vi "Convert Annulus to ROI for Overlay.vi"(8 "error in (no error)":errorcluster, 11 "Mask ROI In":T1={"left annulus"={"Center X"=929, "Center Y"=663, "Inner Radius"=200, "Outer Radius"=405, "Start Angle"=90.0, "End Angle"=180.0}, "right annulus"={"Center X"=929, "Center Y"=663, "Inner Radius"=200, "Outer Radius"=405, "Start Angle"=90.0, "End Angle"=180.0}, "Threshold Range"={"Lower value"=106.82432432432432, "Upper value"=255.0}, "[Avg BG]"=[], "Number of Sectors"=0, "Left ROI"={"Global Rectangle"=[], "Contours"=[]}, "Right ROI"={"Global Rectangle"=[], "Contours"=[]}, "Left Start Angle Duty Cycle"=0.0, "Left End Angle Duty Cycle"=0.0, "Right End Angle Duty Cycle"=0.0, "Right Start Angle Duty Cycle"=0.0, "[Sector ROIs]"=[], "Consecutive Sector Threshold"=0} {"[Sector ROIs]"."Contours"."Type" items=["No Selection", "Point", "Line", "Rectangle", "Oval", "Polygon", "Freehand Region", "Annulus", "Unused2", "Unused3", "Broken Line", "Freehand Line", "Rotated Rectangle"]; "Right ROI"."Contours"."Type" items=["No Selection", "Point", "Line", "Rectangle", "Oval", "Polygon", "Freehand Region", "Annulus", "Unused2", "Unused3", "Broken Line", "Freehand Line", "Rotated Rectangle"]; "Left ROI"."Contours"."Type" items=["No Selection", "Point", "Line", "Rectangle", "Oval", "Polygon", "Freehand Region", "Annulus", "Unused2", "Unused3", "Broken Line", "Freehand Line", "Rotated Rectangle"]; "Threshold Range"."Upper value" min=0.0 max=255.0 scale=0.0..255.0; "Threshold Range"."Lower value" min=0.0 max=255.0 scale=0.0..255.0; "right annulus"."End Angle" format="%.2f"; "right annulus"."Start Angle" format="%.2f"; "right annulus"."Center X" scale=0.0..1024.0; "left annulus"."End Angle" format="%.2f"; "left annulus"."Start Angle" format="%.2f"; "left annulus"."Center X" scale=0.0..1024.0}) -> (0 "error out":errorcluster, 3 "Mask ROI Out":T1={"left annulus"={"Center X"=929, "Center Y"=663, "Inner Radius"=200, "Outer Radius"=405, "Start Angle"=90.0, "End Angle"=180.0}, "right annulus"={"Center X"=929, "Center Y"=663, "Inner Radius"=200, "Outer Radius"=405, "Start Angle"=90.0, "End Angle"=180.0}, "Threshold Range"={"Lower value"=106.82432432432432, "Upper value"=255.0}, "[Avg BG]"=[0, 0, 0, 0, 0, 0, 0, 0, 0, 0, 0, 0, 0, 0, 0, 0, 0, 0, 0, 0, 0, 0, 0, 0, 0, 0, 0, 0, 0, 0, 0, 0], "Number of Sectors"=0, "Left ROI"={"Global Rectangle"=[], "Contours"=[]}, "Right ROI"={"Global Rectangle"=[], "Contours"=[]}, "Left Start Angle Duty Cycle"=0.0, "Left End Angle Duty Cycle"=0.0, "Right End Angle Duty Cycle"=0.0, "Right Start Angle Duty Cycle"=0.0, "[Sector ROIs]"=[], "Consecutive Sector Threshold"=0} {"[Sector ROIs]"."Contours"."Type" items=["No Selection", "Point", "Line", "Rectangle", "Oval", "Polygon", "Freehand Region", "Annulus", "Unused2", "Unused3", "Broken Line", "Freehand Line", "Rotated Rectangle"]; "Right ROI"."Contours"."Type" items=["No Selection", "Point", "Line", "Rectangle", "Oval", "Polygon", "Freehand Region", "Annulus", "Unused2", "Unused3", "Broken Line", "Freehand Line", "Rotated Rectangle"]; "Left ROI"."Contours"."Type" items=["No Selection", "Point", "Line", "Rectangle", "Oval", "Polygon", "Freehand Region", "Annulus", "Unused2", "Unused3", "Broken Line", "Freehand Line", "Rotated Rectangle"]; "Threshold Range"."Upper value" min=0.0 max=255.0 scale=0.0..255.0; "Threshold Range"."Lower value" min=0.0 max=255.0 scale=0.0..255.0; "right annulus"."End Angle" format="%.2f"; "right annulus"."Start Angle" format="%.2f"; "right annulus"."Center X" scale=0.0..1024.0; "left annulus"."End Angle" format="%.2f"; "left annulus"."Start Angle" format="%.2f"; "left annulus"."Center X" scale=0.0..1024.0})   [LabVIEW 2013]
uses:
  Image Processing/Mask ROI Cluster.ctl
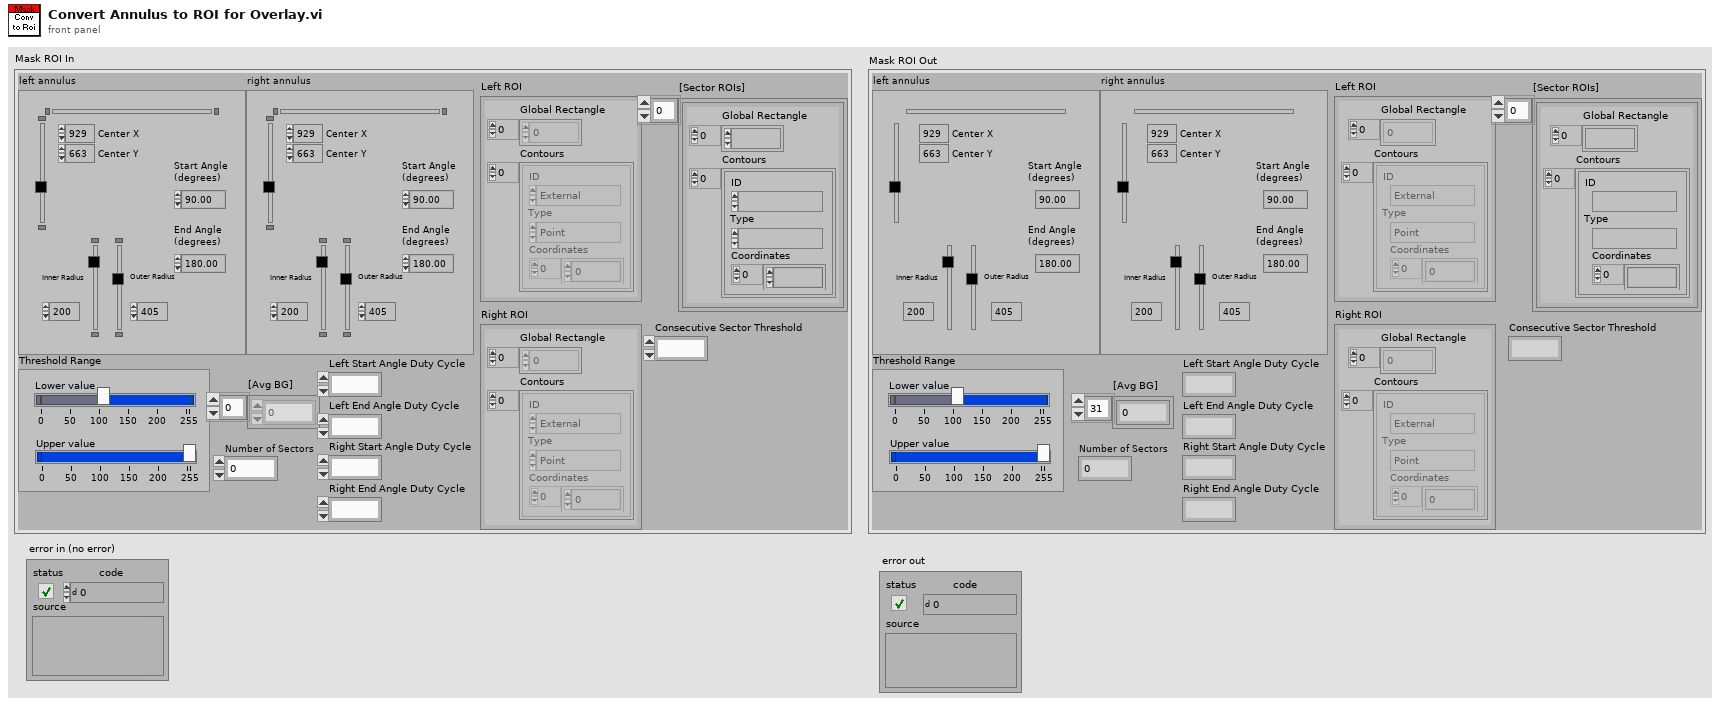
[diagram p1: front panel]
types:
  T1 = typedef "Mask ROI Cluster.ctl" = cluster{"left annulus":T2, "right annulus":T2, "Threshold Range":cluster{"Lower value":dbl, "Upper value":dbl}, "[Avg BG]":u8[], "Number of Sectors":u8, "Left ROI":T3, "Right ROI":T3, "Left Start Angle Duty Cycle":fxp<+,8,0>, "Left End Angle Duty Cycle":fxp<+,8,0>, "Right End Angle Duty Cycle":fxp<+,8,0>, "Right Start Angle Duty Cycle":fxp<+,8,0>, "[Sector ROIs]":T3[], "Consecutive Sector Threshold":u8}
  T2 = typedef "IMAQ Circle" = cluster{"Center X":i32, "Center Y":i32, "Inner Radius":i32, "Outer Radius":i32, "Start Angle":dbl, "End Angle":dbl}
  T3 = typedef "ROI Descriptor" = cluster{"Global Rectangle":i32[], "Contours":cluster{"ID":enum32{"External", "Internal"}, "Type":u32, "Coordinates":i32[]}[]}
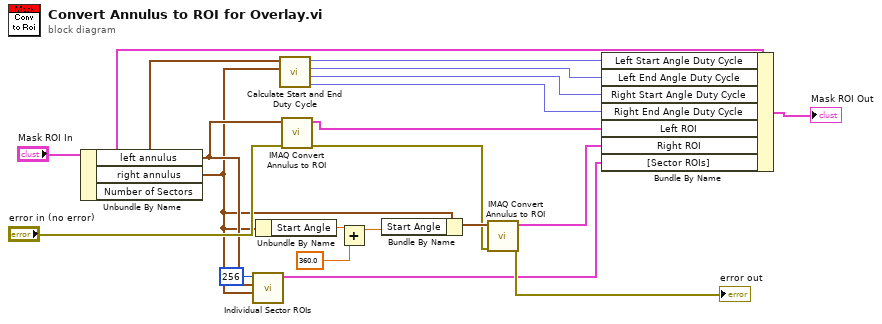
[diagram p0: block diagram]
diagram:
  n1 = Unbundle By Name("Mask ROI In") -> ("left annulus"=w3:T2, "right annulus"=w2:T2)  [unwired: 1 out]
  n2 = call "Individual Sector ROIs.vi"("right annulus"=w2, "left annulus"=w3, "Number of Sectors"=u16 256) -> ("Sector ROIs"=w4:T3[])  [unwired: 8 in]
  n3 = Unbundle By Name(w2) -> ("Start Angle"=w19:dbl)
  n4 = call "Calculate Start and End Duty Cycle.vi"("right annulus"=w2, "left annulus"=w3) -> ("Right End Angle Duty Cycle"=w5:fxp<+,8,0>, "Right Start Angle Duty Cycle"=w6:fxp<+,8,0>, "Left End Angle Duty Cycle"=w7:fxp<+,8,0>, "Left Start Angle Duty Cycle"=w8:fxp<+,8,0>)  [unwired: 6 in]
  n5 = call "IMAQ Convert Annulus to ROI"("error in (no error)"="error in (no error)", "Annulus"=w3) -> ("error out"=w10:errorcluster, "ROI Descriptor"=w14:T3)  [unwired: 7 in]
  n6 = Add(x=w19, y=360.0) -> (x+y=w17:dbl)
  n7 = Bundle By Name(cluster=w2, "Start Angle"=w17) -> (w16:T2)
  n8 = call "IMAQ Convert Annulus to ROI"("error in (no error)"=w10, "Annulus"=w16) -> ("error out"=→"error out":errorcluster, "ROI Descriptor"=w13:T3)  [unwired: 7 in]
  n9 = Bundle By Name(cluster="Mask ROI In", "Left Start Angle Duty Cycle"=w8, "Left End Angle Duty Cycle"=w7, "Right Start Angle Duty Cycle"=w6, "Right End Angle Duty Cycle"=w5, "Left ROI"=w14, "Right ROI"=w13, "[Sector ROIs]"=w4) -> (→"Mask ROI Out":T1)
